vi "Set MenuItemList.vi"(8 "error in (no error)":errorcluster, 10 "MenuItemList":string[](array[string])=["<No Items Defined>"], 11 "MenuCol in":refnum<class "MenuCol.lvclass">) -> (0 "error out":errorcluster, 3 "MenuCol out":refnum<class "MenuCol.lvclass">)   [LabVIEW 2013, in "MenuCol.lvclass"]
uses:
  MenuCol.lvclass
  MenuCol.lvclass/MenuCol.ctl
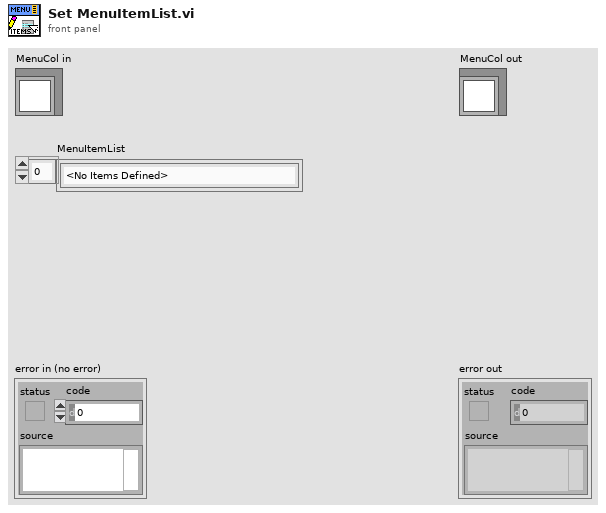
[diagram p1: front panel]
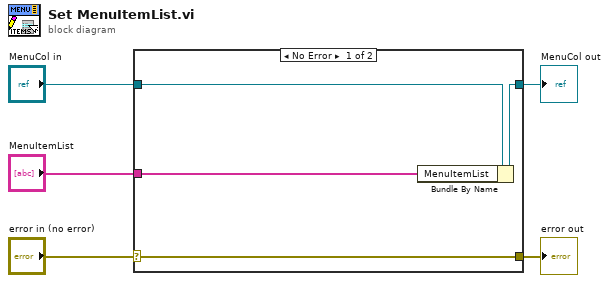
[diagram p0: block diagram]
diagram:
  n1 = case shown="No Error" "error in (no error)" {
    selector: "error in (no error)" -> [w9 w10]
    tunnel: [w9 w10] -> w4
    tunnel: [w7 w11] -> w2
    tunnel: "MenuCol in" -> [w8 w11]
    tunnel: "MenuItemList" -> [w6 _]
    frame No Error {
      n2 = Bundle By Name(cluster=w8, "MenuItemList"=w6) -> (w7:refnum<class "MenuCol.lvclass">)
    }
    frame Error {
    }
  }
  "error out" <- w4
  "MenuCol out" <- w2
